vi "file_pre_process.vi"(6 "Sensor Lookup Indices":i32[](array[numeric]), 8 "error in (no error)":errorcluster, 9 "Pkt Size":i32, 10 "Gains":dbl[](array[numeric]), 11 "Path":path) -> (0 "error out":errorcluster, 2 "Sensor_Tare":dbl[][](array[numeric]), 3 "Sensor Output - Position (mm)":dbl[][][](array[numeric]))   [LabVIEW 2018]
panel:
  out "No. Packets":dbl
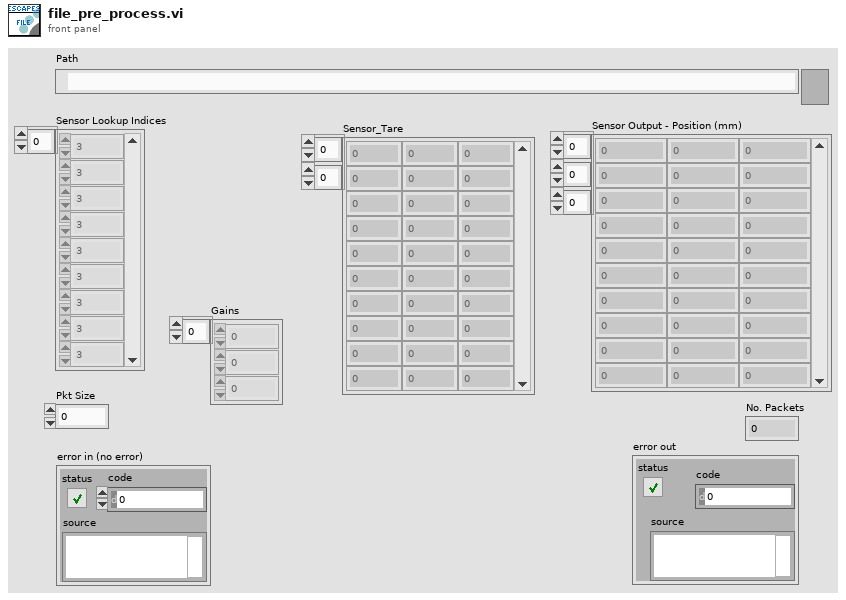
[diagram p1: front panel]
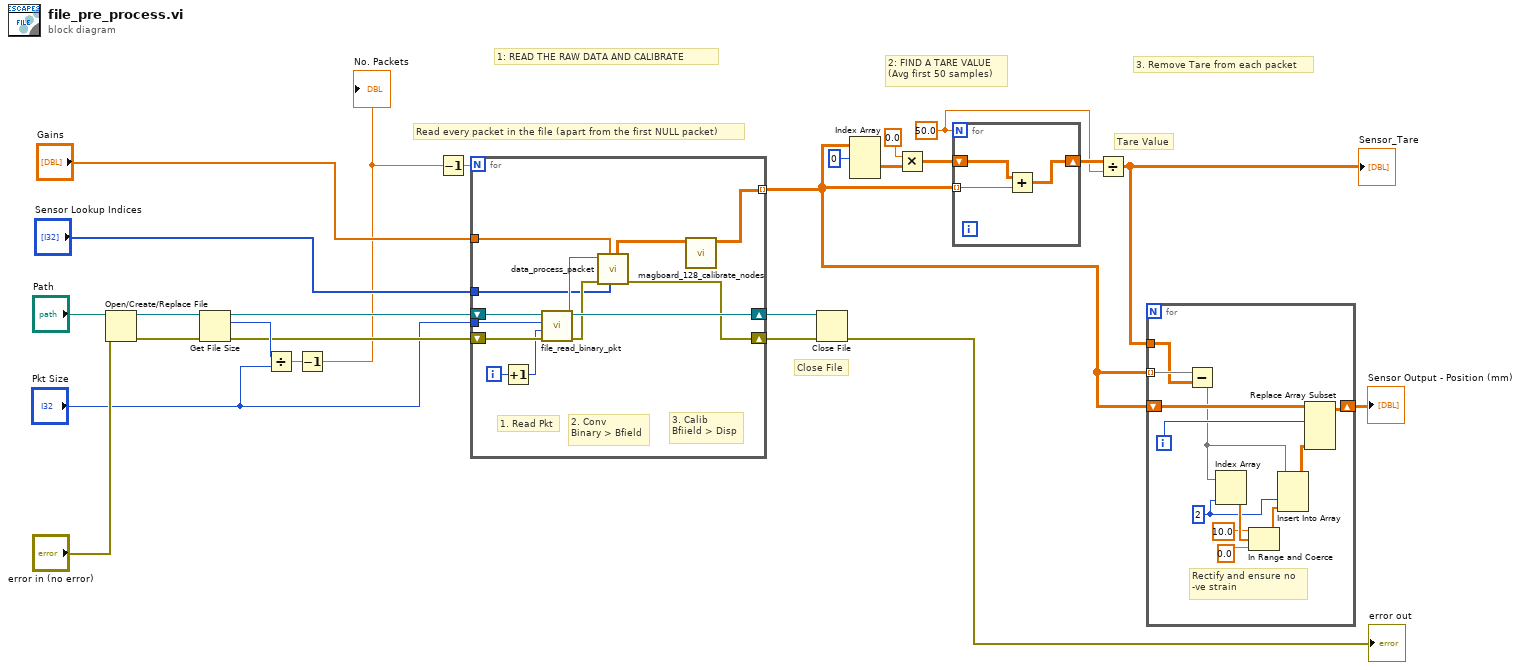
[diagram p0: block diagram]
diagram:
  w7 = 50.0
  # "3. Remove Tare from each packet"
  # "Close File"
  # "Tare Value"
  # "2: FIND A TARE VALUE\n(Avg first 50 samples)"
  # "1: READ THE RAW DATA AND CALIBRATE"
  # "Read every packet in the file (apart from the first NULL packet)"
  n1 = Open/Create/Replace File(file path (use dialog)="Path", error in="error in (no error)") -> (refnum out=w23:refnum<file>, error out=w22:errorcluster)  [unwired: 4 in, 1 out]
  n2 = Get File Size(file=w23, error in=w22) -> (refnum out=w18:refnum<file>, size (in bytes)=w20:i64, 0:w16:errorcluster)
  n3 = Divide(x=w20, y="Pkt Size") -> (x/y=w21:dbl)
  n4 = Decrement(x=w21) -> (x-1=w13:dbl)
  "No. Packets" <- w13
  n5 = Decrement(x=w13) -> (x-1=w14:dbl)
  n6 = for {
    N: w14 -> [_]
    tunnel: "Pkt Size" -> [w37]
    shift-right: [w36] -> w6
    shift-left: w18 -> [w38]
    shift-right: [w31] -> w5
    shift-left: w16 -> [w35]
    tunnel: "Gains" -> [w30]
    tunnel: "Sensor Lookup Indices" -> [w29]
    tunnel: [w26] -> w3 mode=indexing
    i -> [w27]
    # "3. Calib\nBfiield > Disp"
    # "2. Conv\nBinary > Bfield"
    # "1. Read Pkt"
    n7 = Increment(x=w27) -> (x+1=w28:i32)
    n8 = call "file_read_binary_pkt.vi"("error in (no error)"=w35, "Packet No."=w28, "Pkt Size(bytes)"=w37, "Byte Stream File in"=w38) -> ("error out"=w33:errorcluster, "Packet"=w34:string, "Byte Stream File out"=w36:refnum<file>)  [unwired: 4 in, 1 out]
    n9 = call "data_process_packet.vi"("Sensor Lookup Indices"=w29, "Gains"=w30, "error in (no error)"=w33, "Binary Input Data"=w34) -> ("error out"=w31:errorcluster, "Sensors (uT)"=w32:dbl[][])  [unwired: 3 in, 3 out]
    n10 = call "magboard_128_calibrate_nodes.vi"("Sensor Input (mT)"=w32) -> ("Sensor Output - Position (mm)"=w26:dbl[][])  [unwired: 10 in]
  }
  n11 = Close File(refnum=w6, error in=w5) -> (error out=→"error out":errorcluster)  [unwired: 1 out]
  n12 = Index Array(array=w3, index (dim 0)=0 ("index (page)")) -> (element=w10:dbl[][])  [unwired: 2 in]
  n13 = Multiply(x=0.0, y=w10) -> (x*y=w11:dbl[][])
  n14 = for {
    N: w7 -> [_]
    tunnel: w3 -> [w40] mode=indexing
    shift-right: [w39] -> w8
    shift-left: w11 -> [w41]
    n15 = Add(x=w41, y=w40) -> (x+y=w39:dbl[][])
  }
  n16 = Divide(x=w8, y=w7) -> (x/y=w2:dbl[][])
  "Sensor_Tare" <- w2
  n17 = for {
    tunnel: w3 -> [w52] mode=indexing
    tunnel: w2 -> [w51]
    shift-right: [w49] -> w1
    shift-left: w3 -> [w53]
    i -> [w50]
    w42 = 2 ("disabled index (col)")
    # "Rectify and ensure no\n-ve strain"
    n18 = Subtract(x=w52, y=w51) -> (x-y=w43:dbl[][])
    n19 = Index Array(array=w43, index (col)=w42) -> (element=w48:dbl[])  [unwired: 1 in]
    n20 = In Range and Coerce(upper limit=10.0, x=w48, lower limit=0.0) -> (coerced(x)=w44:dbl[])  [unwired: 1 out]
    n21 = Insert Into Array(array=w43, index (col)=w42, new element=w44) -> (w45:dbl[][])  [unwired: 1 in]
    n22 = Replace Array Subset(array=w53, new element=w45, index (dim 0)=w50) -> (w49:dbl[][][])  [unwired: 2 in]
  }
  "Sensor Output - Position (mm)" <- w1
